vi "SortClicks.vi"(7 "Table History ref":refnum<vi>, 8 "error in (no error)":errorcluster, 10 "ClickEvent in":T3, 11 "Col array in":refnum<class "Column.lvclass">[](array[class])) -> (0 "error out":errorcluster, 1 "Row Type":T2, 2 "Click out":T1, 3 "Col array out":refnum<class "Column.lvclass">[](array[class]), 4 "Update HWI?":bool, 5 "withinData?":bool=TRUE)   [LabVIEW 2013]
doc: "Specialize click-sorting for SetList Table. The case structure was forcing the Table control event loop within the main SetList program to be very large, so I've moved the click-sorting within this SubVI.\n\nFor an overview of how clicks are sorted, see the additional documentation (or read comments)."
uses:
  TypeDefs/ClickEvent.ctl
  <vilib>/Utility/miscctls.llb/LVPoint32TypeDef.ctl
  TypeDefs/TableHistory.ctl
  TypeDefs/TableArray.ctl
  ColumnVIs/Column/Column.lvclass
  TypeDefs/RowType.ctl
  TypeDefs/ClickReturn.ctl
  <vilib>/Utility/miscctls.llb/LVRowAndColumnTypeDef.ctl
  Globals/DisabledColorGlobal.vi
panel:
  out "disabled?":bool
  # "Change this typedef if LabVIEW changes what is provided on click event!"
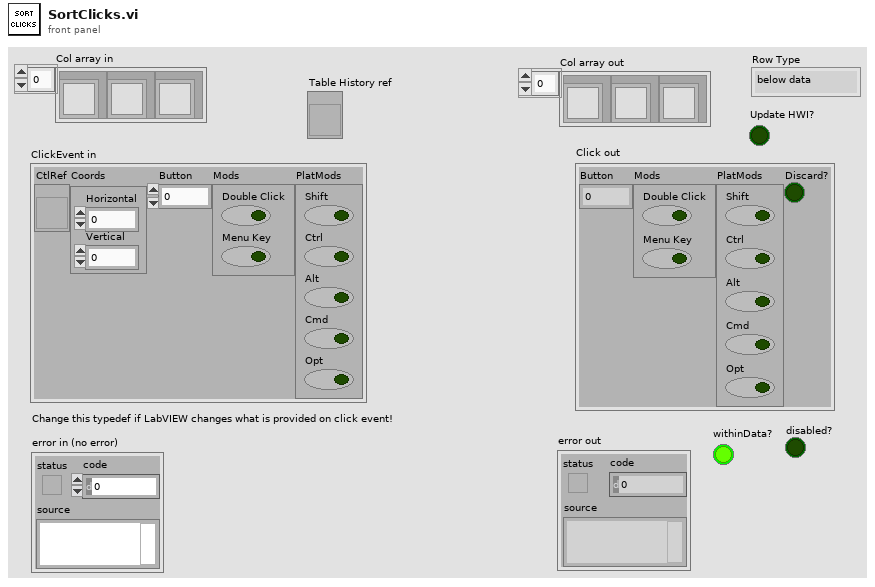
[diagram p1: front panel]
types:
  T1 = typedef "ClickReturn.ctl" = cluster{"Button":u16, "Mods":cluster{"Double Click":bool, "Menu Key":bool}, "PlatMods":cluster{"Shift":bool, "Ctrl":bool, "Alt":bool, "Cmd":bool, "Opt":bool}, "Discard?":bool}
  T2 = typedef "RowType.ctl" = enum16{"below data", "within data", "column header", "first row"}
  T3 = typedef "ClickEvent.ctl" = cluster{"CtlRef":refnum<vi>, "Coords":T4, "Button":u16, "Mods":cluster{"Double Click":bool, "Menu Key":bool}, "PlatMods":cluster{"Shift":bool, "Ctrl":bool, "Alt":bool, "Cmd":bool, "Opt":bool}}
  T4 = typedef "LVPoint32TypeDef.ctl" = cluster{"Horizontal":i32, "Vertical":i32}
  T5 = cluster{"Shift":bool, "Ctrl":bool, "Alt":bool, "Cmd":bool, "Opt":bool}
  T6 = typedef "LVRowAndColumnTypeDef.ctl" = cluster{"Row":i32, "Column":i32}
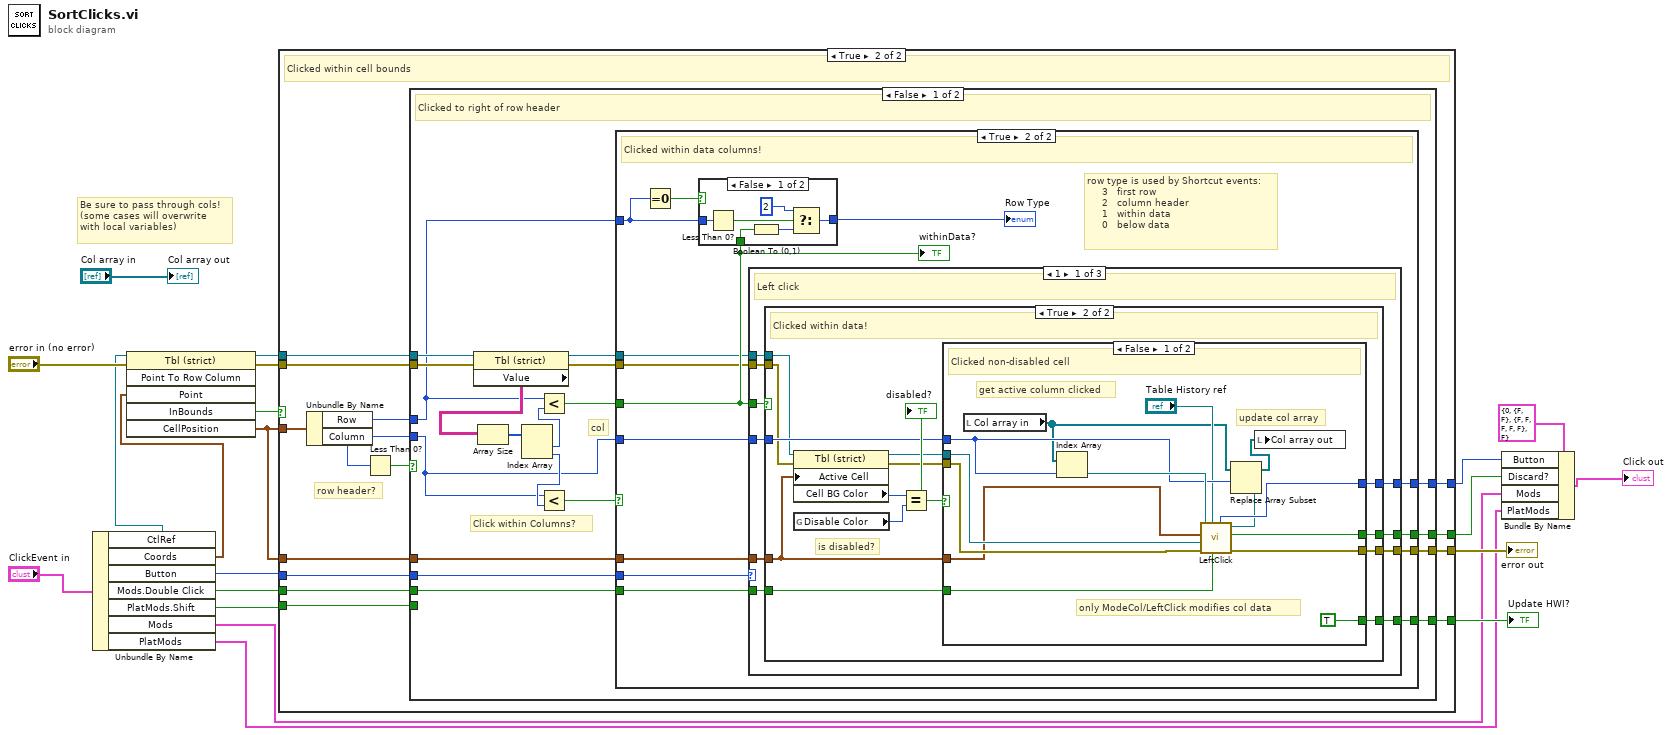
[diagram p0: block diagram]
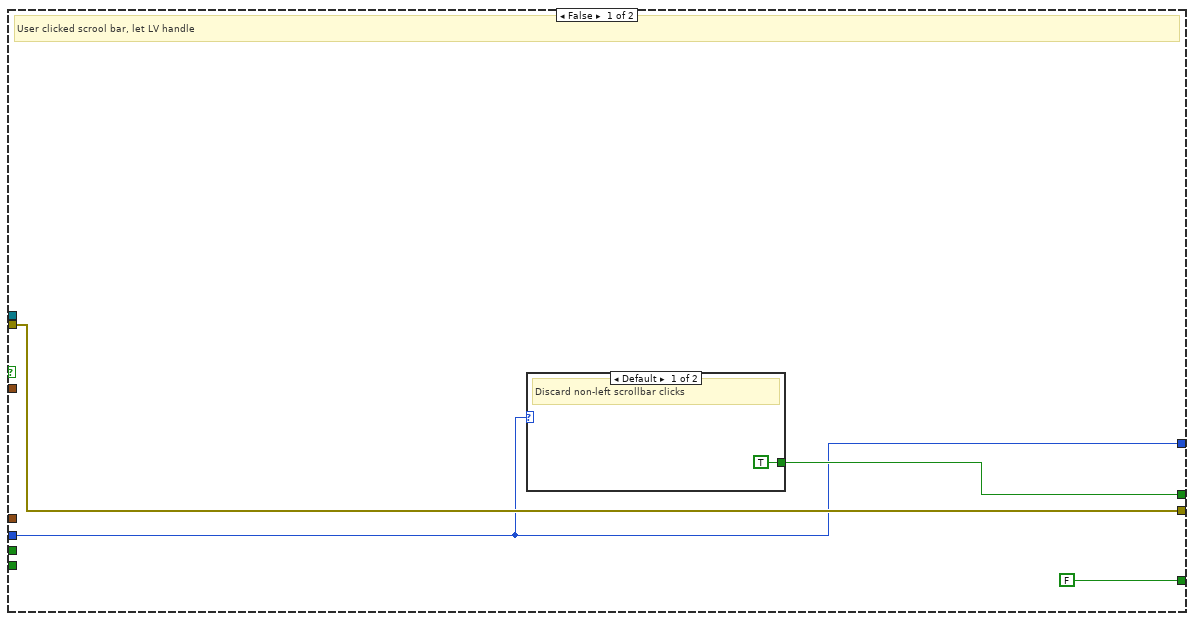
[diagram p2: hidden frame]
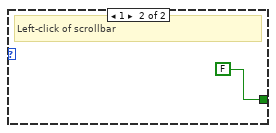
[diagram p3: hidden frame]
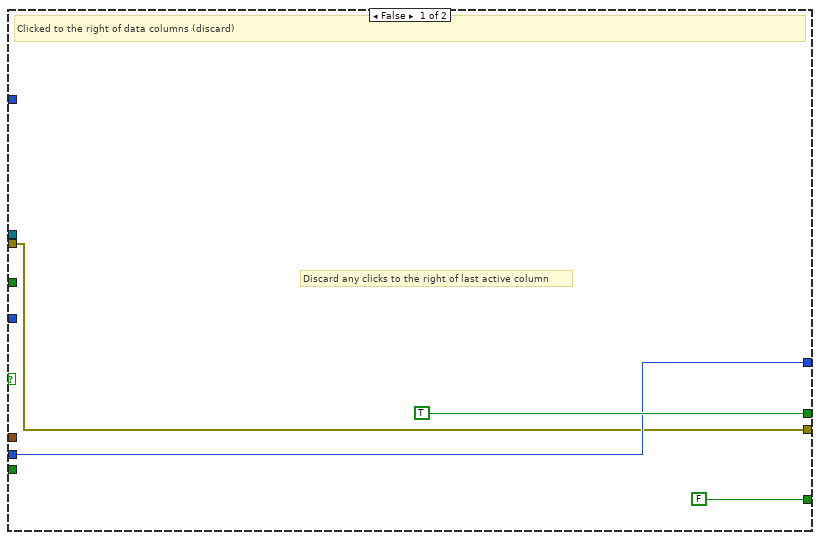
[diagram p4: hidden frame]
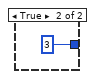
[diagram p5: hidden frame]
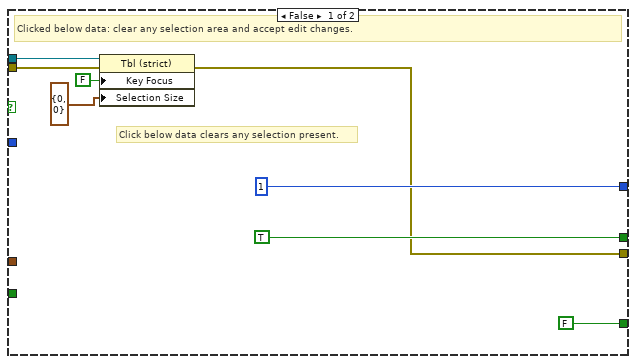
[diagram p6: hidden frame]
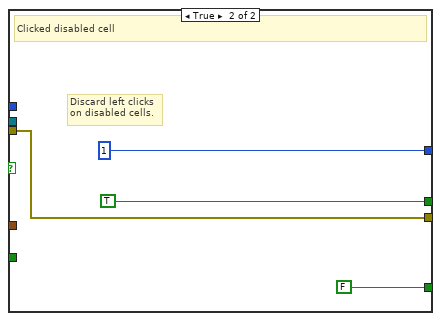
[diagram p7: hidden frame]
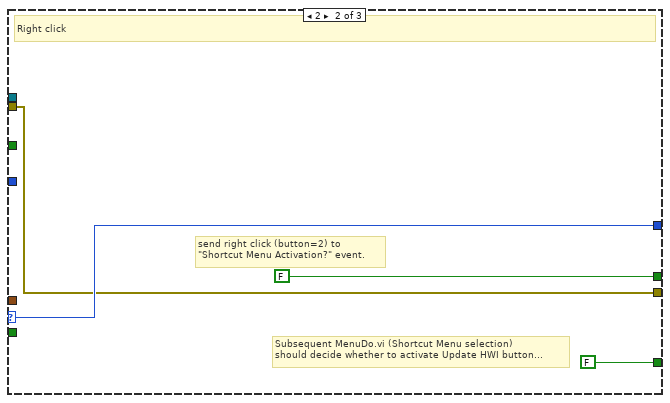
[diagram p8: hidden frame]
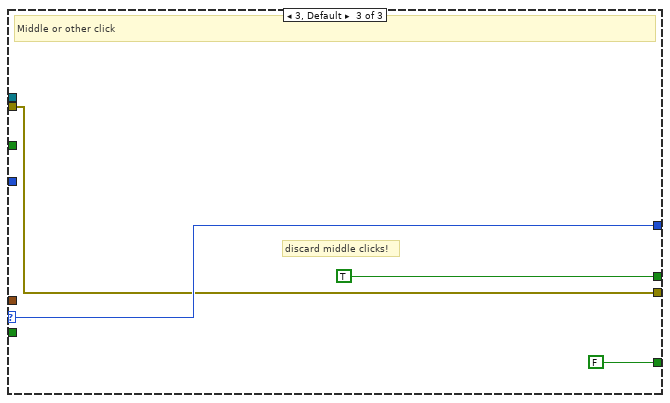
[diagram p9: hidden frame]
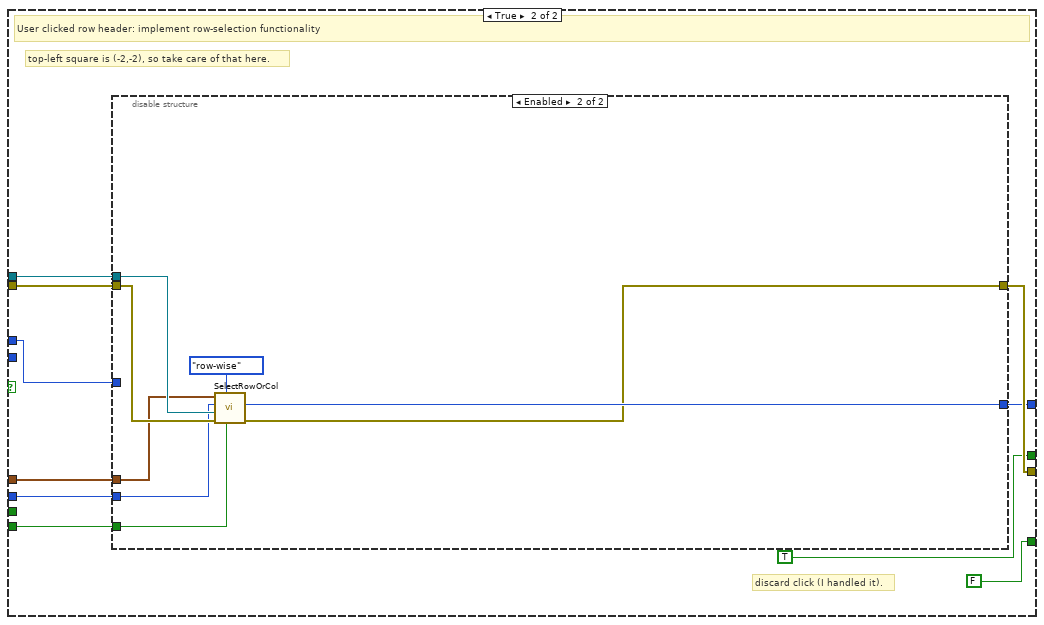
[diagram p10: hidden frame]
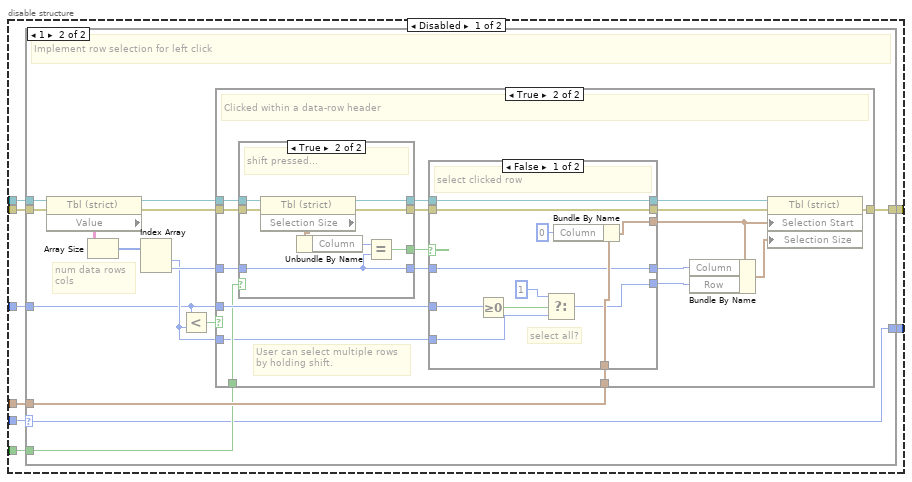
[diagram p11: hidden frame]
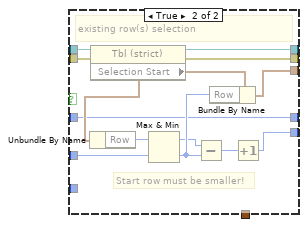
[diagram p14: hidden frame]
diagram:
  # "Be sure to pass through cols!\n(some cases will overwrite \nwith local variables)"
  n1 = Unbundle By Name("ClickEvent in") -> ("CtlRef"=w15:refnum<vi>, "Coords"=w11:T4, "Button"=w12:u16, "Mods.Double Click"=w14:bool, "PlatMods.Shift"=w13:bool, "Mods"=w2:cluster{"Double Click":bool, "Menu Key":bool}, "PlatMods"=w1:T5)
  n2 = invoke class="Tbl (strict)" method="Point To Row Column"(reference=w15, error in="error in (no error)", "Point"=w11) -> (reference out=w20:refnum<vi>, error out=w19:errorcluster, "InBounds"=w18:bool, "CellPosition"=w5:T6)  [unwired: 3 in, 2 out]
  n3 = case shown="True" w18 {
    tunnel: [w24 w38] -> w3
    tunnel: w5 -> [_ w40]
    tunnel: w19 -> [w23 w37]
    tunnel: w20 -> [_ w36]
    tunnel: w12 -> [w21 w33]
    tunnel: w14 -> [_ w30]
    tunnel: w5 -> [_ w31]
    tunnel: [w23 w29] -> w10
    tunnel: [w21 w32] -> w7
    tunnel: w13 -> [_ w28]
    tunnel: [FALSE w27] -> w6
    frame False {
      # "User clicked scrool bar, let LV handle"
      n4 = case shown="Default" w21 {
        tunnel: [TRUE FALSE] -> w24
        frame Default {
          # "Discard non-left scrollbar clicks"
        }
        frame 1 {
          # "Left-click of scrollbar"
        }
      }
    }
    frame True {
      # "row header?"
      # "Clicked within cell bounds"
      n5 = Unbundle By Name(w40) -> ("Row"=w35:i32, "Column"=w34:i32)
      n6 = Less Than 0?(x=w34) -> (x < 0?=w39:bool)
      n7 = case shown="False" w39 {
        tunnel: [w51 TRUE] -> w38
        tunnel: w35 -> [w41 w149]
        tunnel: w37 -> [w54 w151]
        tunnel: w36 -> [w55 w150]
        tunnel: w34 -> [w44 _]
        tunnel: w33 -> [w52 w146]
        tunnel: [w49 w144] -> w32
        tunnel: w31 -> [w46 w148]
        tunnel: w30 -> [w45 _]
        tunnel: [w43 w152] -> w29
        tunnel: w28 -> [_ w147]
        tunnel: [w42 FALSE] -> w27
        frame False {
          # "col"
          # "Click within Columns?"
          # "Clicked to right of row header"
          n8 = property class="Tbl (strict)"(reference=w55, error in=w54) -> (reference out=w48:refnum<vi>, error out=w47:errorcluster, "Value"=w59:string[][])
          n9 = Array Size(array=w59) -> (size(s)=w58:i32[])
          n10 = Index Array(array=w58) -> (element #1=w57:i32, element #2=w56:i32)  [unwired: 2 in]
          n11 = Less?(x=w41, y=w57) -> (x < y?=w50:bool)
          n12 = Less?(x=w44, y=w56) -> (x < y?=w53:bool)
          n13 = case shown="True" w53 {
            tunnel: w50 -> [_ w71]
            tunnel: w52 -> [w62 w77]
            tunnel: [TRUE w76] -> w51
            tunnel: [w62 w75] -> w49
            tunnel: w48 -> [_ w69]
            tunnel: w47 -> [w61 w68]
            tunnel: w46 -> [_ w70]
            tunnel: w45 -> [_ w74]
            tunnel: w44 -> [_ w73]
            tunnel: [w61 w72] -> w43
            tunnel: w41 -> [_ w67]
            tunnel: [FALSE w64] -> w42
            frame False {
              # "Discard any clicks to the right of last active column"
              # "Clicked to the right of data columns (discard)"
            }
            frame True {
              # "row type is used by Shortcut events:\n     3   first row\n     2   column header\n     1   within data\n     0   below data"
              # "Clicked within data columns!"
              n14 = Equal To 0?(x=w67) -> (x = 0?=w66:bool)
              n15 = case shown="False" w66 {
                tunnel: [w81 i16 3] -> w65
                tunnel: w71 -> [w80 _]
                tunnel: w67 -> [w78 _]
                frame False {
                  n16 = Less Than 0?(x=w78) -> (x < 0?=w79:bool)
                  n17 = Boolean To (0,1)(Boolean=w80) -> (0, 1=w82:i16)
                  n18 = Select(t=i16 2, s=w79, f=w82) -> (s? t:f=w81:i16)
                }
                frame True {
                }
              }
              "Row Type" <- w65
              n19 = case shown="1" w77 {
                selector: w77 -> [_ w137 w141]
                tunnel: [w93 FALSE TRUE ("Discard?")] -> w76
                tunnel: w71 -> [w94 _ _]
                tunnel: [w92 w137 w141] -> w75
                tunnel: w70 -> [w91 _ _]
                tunnel: w74 -> [w90 _ _]
                tunnel: w73 -> [w89 _ _]
                tunnel: [w88 w136 w140] -> w72
                tunnel: w69 -> [w87 _ _]
                tunnel: w68 -> [w86 w136 w140]
                tunnel: [w85 FALSE FALSE] -> w64
                frame 1 {
                  # "Left click"
                  n20 = case shown="True" w94 {
                    tunnel: [TRUE w113] -> w93
                    tunnel: [u16 1 w112] -> w92
                    tunnel: w91 -> [_ w106]
                    tunnel: w90 -> [_ w111]
                    tunnel: w89 -> [_ w110]
                    tunnel: [w97 w107] -> w88
                    tunnel: w87 -> [w99 w105]
                    tunnel: w86 -> [w98 w104]
                    tunnel: [FALSE w103] -> w85
                    frame False {
                      # "Click below data clears any selection present."
                      # "Clicked below data: clear any selection area and accept edit changes."
                      n21 = property class="Tbl (strict)"(reference=w99, error in=w98, "Key Focus"=FALSE, "Selection Size"=T6 {"Row"=0, "Column"=0}) -> (error out=w97:errorcluster)  [unwired: 1 out]
                    }
                    frame True {
                      # "is disabled?"
                      # "Clicked within data!"
                      n22 = property class="Tbl (strict)"(reference=w105, error in=w104, "Active Cell"=w106) -> (reference out=w109:refnum<vi>, error out=w108:errorcluster, "Cell BG Color"=w116:u32)
                      n23 = global read "DisabledColorGlobal.vi" "Disable Color"() -> (w115:u32)
                      n24 = Equal?(x=w116, y=w115) -> (x = y?=w114:bool)
                      "disabled?" <- w114
                      n25 = case shown="False" w114 {
                        tunnel: [w130 TRUE] -> w113
                        tunnel: [w127 u16 1] -> w112
                        tunnel: w111 -> [w121 _]
                        tunnel: w110 -> [w125 _]
                        tunnel: w109 -> [w124 _]
                        tunnel: w108 -> [w123 w132]
                        tunnel: [w128 w132] -> w107
                        tunnel: w106 -> [w122 _]
                        tunnel: [TRUE FALSE] -> w103
                        frame False {
                          # "only ModeCol/LeftClick modifies col data"
                          # "update col array"
                          # "get active column clicked"
                          # "Clicked non-disabled cell"
                          n26 = local read "Col array in"() -> (w117:refnum<class "Column.lvclass">[])
                          n27 = Index Array(array=w117, index=w125) -> (element=w129:refnum<class "Column.lvclass">)
                          n28 = call-dynamic "LeftClick.vi"("Double Click"=w121, "Table History ref"="Table History ref", "error in (no error)"=w123, "Table CtlRef In"=w124, "Cell Position"=w122, "Column in"=w129) -> ("error out"=w128:errorcluster, "Discard?"=w130:bool, "Column out"=w126:refnum<class "Column.lvclass">, "Button"=w127:u16)  [unwired: 1 in, 1 out]
                          n29 = Replace Array Subset(array=w117, new element=w126, index=w125) -> (w118:refnum<class "Column.lvclass">[])
                          n30 = local write "Col array out"(w118) -> ()
                        }
                        frame True {
                          # "Discard left clicks\non disabled cells."
                          # "Clicked disabled cell"
                        }
                      }
                    }
                  }
                }
                frame 2 {
                  # "Subsequent MenuDo.vi (Shortcut Menu selection)\nshould decide whether to activate Update HWI button..."
                  # "send right click (button=2) to \n\"Shortcut Menu Activation?\" event."
                  # "Right click"
                }
                frame 3, Default {
                  # "discard middle clicks!"
                  # "Middle or other click"
                }
              }
              "withinData?" <- w71
            }
          }
        }
        frame True {
          # "discard click (I handled it)."
          # "top-left square is (-2,-2), so take care of that here."
          # "User clicked row header: implement row-selection functionality"
          n31 = disable-structure shown="Enabled" {
            disable-tunnel: [w160 w235] -> w152
            disable-tunnel: w151 -> [w159 w238]
            disable-tunnel: w150 -> [w158 w239]
            disable-tunnel: w149 -> [w157 _]
            disable-tunnel: w148 -> [w156 w233]
            disable-tunnel: w147 -> [w155 w232]
            disable-tunnel: w146 -> [w154 w237]
            disable-tunnel: [w153 w236] -> w144
            frame Disabled {
              n32 = case shown="1" w154 {
                selector: w154 -> [w161 w167]
                tunnel: [w162 w176] -> w160
                tunnel: w159 -> [w162 w175]
                tunnel: w158 -> [_ w174]
                tunnel: w157 -> [_ w164]
                tunnel: w156 -> [_ w169]
                tunnel: w155 -> [_ w168]
                tunnel: [w161 w167] -> w153
                frame Default {
                }
                frame 1 {
                  # "num data rows\ncols"
                  # "Implement row selection for left click"
                  n33 = property class="Tbl (strict)"(reference=w174, error in=w175) -> (reference out=w171:refnum<vi>, error out=w170:errorcluster, "Value"=w173:string[][])
                  n34 = Array Size(array=w173) -> (size(s)=w172:i32[])
                  n35 = Index Array(array=w172) -> (element #1=w165:i32, element #2=w166:i32)  [unwired: 2 in]
                  n36 = Less?(x=w164, y=w165) -> (x < y?=w163:bool)
                  n37 = case shown="True" w163 {
                    tunnel: [w177 w195] -> w176
                    tunnel: w171 -> [_ w194]
                    tunnel: w170 -> [w177 w193]
                    tunnel: w164 -> [_ w187]
                    tunnel: w169 -> [_ w186]
                    tunnel: w168 -> [_ w180]
                    tunnel: w165 -> [_ w179]
                    tunnel: w166 -> [_ w178]
                    frame False {
                      # "ignore row clicks below data!"
                    }
                    frame True {
                      # "User can select multiple rows\nby holding shift."
                      # "Clicked within a data-row header"
                      n38 = case shown="True" w180 {
                        selector: w180 -> [w223 _]
                        tunnel: w194 -> [w222 w231]
                        tunnel: w193 -> [w221 w230]
                        tunnel: [w221 w229] -> w190
                        tunnel: [w222 w228] -> w192
                        tunnel: w178 -> [w220 w224]
                        tunnel: [w223 w225] -> w188
                        tunnel: [w220 w224] -> w185
                        frame False {
                        }
                        frame True {
                          # "shift pressed..."
                          n39 = property class="Tbl (strict)"(reference=w231, error in=w230) -> (reference out=w228:refnum<vi>, error out=w229:errorcluster, "Selection Size"=w227:T6)
                          n40 = Unbundle By Name(w227) -> ("Column"=w226:i32)
                          n41 = Equal?(x=w226, y=w224) -> (x = y?=w225:bool)
                        }
                      }
                      n42 = case shown="False" w188 {
                        tunnel: w192 -> [w206 w219]
                        tunnel: [w206 w218] -> w191
                        tunnel: w190 -> [w205 w217]
                        tunnel: [w205 w216] -> w189
                        tunnel: w187 -> [w200 w214]
                        tunnel: [w203 w213] -> w183
                        tunnel: w186 -> [w204 _]
                        tunnel: w185 -> [w201 w208]
                        tunnel: [w201 w208] -> w184
                        tunnel: [w198 w207] -> w181
                        tunnel: w179 -> [w196 _]
                        frame False {
                          # "select all?"
                          # "select clicked row"
                          n43 = Greater Or Equal To 0?(x=w200) -> (x >= 0?=w199:bool)
                          n44 = Select(t=1, s=w199, f=w196) -> (s? t:f=w198:i32)
                          n45 = Bundle By Name(cluster=w204, "Column"=0) -> (w203:T6)
                        }
                        frame True {
                          # "Start row must be smaller!"
                          # "existing row(s) selection"
                          n46 = property class="Tbl (strict)"(reference=w219, error in=w217) -> (reference out=w218:refnum<vi>, error out=w216:errorcluster, "Selection Start"=w209:T6)
                          n47 = Unbundle By Name(w209) -> ("Row"=w215:i32)
                          n48 = Max & Min(x=w215, y=w214) -> (max(x,y)=w211:i32, min(x,y)=w212:i32)
                          n49 = Subtract(x=w211, y=w212) -> (x-y=w210:i32)
                          n50 = Bundle By Name(cluster=w209, "Row"=w212) -> (w213:T6)
                          n51 = Increment(x=w210) -> (x+1=w207:i32)
                        }
                      }
                      n52 = Bundle By Name(cluster=w183, "Column"=w184, "Row"=w181) -> (w182:T6)
                      n53 = property class="Tbl (strict)"(reference=w191, error in=w189, "Selection Start"=w183, "Selection Size"=w182) -> (error out=w195:errorcluster)  [unwired: 1 out]
                    }
                  }
                }
              }
            }
            frame Enabled {
              n54 = call "SelectRowOrCol.vi"("Shift Pressed? (F)"=w232, "Row/Col"=enum16{"row-wise", "col-wise"}."row-wise", "error in"=w238, "Table CtlRef"=w239, "Button (1)"=w237, "CellPosition"=w233) -> ("error out"=w235:errorcluster, "Button"=w236:u16)  [unwired: 4 in]
            }
          }
        }
      }
    }
  }
  "error out" <- w10
  "Update HWI?" <- w6
  n55 = Bundle By Name(cluster=T1 {"Button"=0, "Mods"={"Double Click"=FALSE, "Menu Key"=FALSE}, "PlatMods"={"Shift"=FALSE, "Ctrl"=FALSE, "Alt"=FALSE, "Cmd"=FALSE, "Opt"=FALSE}, "Discard?"=FALSE} ("Click out"), "Button"=w7, "Discard?"=w3, "Mods"=w2, "PlatMods"=w1) -> (→"Click out":T1)
  "Col array out" <- "Col array in"
